vi "Update Preview Image.vi"(0 "Images (Dest)":T1, 2 "Buttons":T3, 3 "error in":errorcluster) -> (6 "Images (Out)":T1, 9 "error out":errorcluster)   [LabVIEW 2011]
uses:
  LCOS Images.ctl
  <vilib>/vision/Image Controls.llb/IMAQ Image.ctl
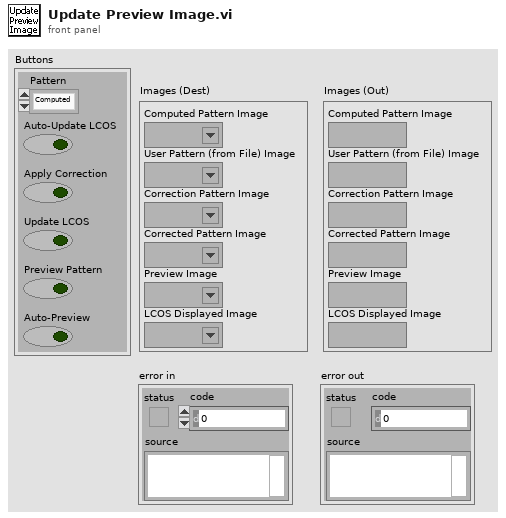
[diagram p1: front panel]
types:
  T1 = typedef "LCOS Images.ctl" = cluster{"Computed Pattern Image":T2, "User Pattern (from File) Image":T2, "Correction Pattern Image":T2, "Corrected Pattern Image":T2, "Preview Image":T2, "LCOS Displayed Image":T2}
  T2 = typedef "IMAQ Image.ctl" = refnum<image>
  T3 = cluster{"Pattern":enum16{"Computed", "From File", "Correction"}, "Auto-Update LCOS":bool, "Apply Correction":bool, "Update LCOS":bool, "Preview Pattern":bool, "Auto-Preview":bool}
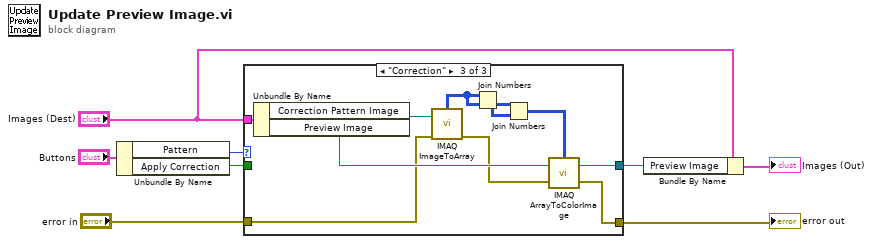
[diagram p0: block diagram]
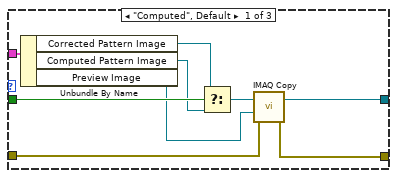
[diagram p2: hidden frame]
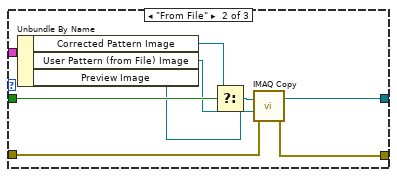
[diagram p3: hidden frame]
diagram:
  n1 = Unbundle By Name("Buttons") -> ("Pattern"=w7:enum16{"Computed", "From File", "Correction"}, "Apply Correction"=w6:bool)
  n2 = case shown="\"Correction\"" w7 {
    tunnel: w6 -> [w16 w25 _]
    tunnel: "Images (Dest)" -> [w17 w26 w36]
    tunnel: "error in" -> [w11 w20 w30]
    tunnel: [w10 w19 w27] -> w3
    tunnel: [w9 w18 w28] -> w1
    frame "Computed", Default {
      n3 = Unbundle By Name(w17) -> ("Corrected Pattern Image"=w15:T2, "Computed Pattern Image"=w14:T2, "Preview Image"=w12:T2)
      n4 = Select(t=w15, s=w16, f=w14) -> (s? t:f=w13:T2)
      n5 = call "IMAQ Copy"("error in (no error)"=w11, "Image Dst"=w12, "Image Src"=w13) -> ("error out"=w9:errorcluster, "Image Dst Out"=w10:T2)  [unwired: 3 in]
    }
    frame "From File" {
      n6 = Unbundle By Name(w26) -> ("Corrected Pattern Image"=w24:T2, "User Pattern (from File) Image"=w23:T2, "Preview Image"=w21:T2)
      n7 = Select(t=w24, s=w25, f=w23) -> (s? t:f=w22:T2)
      n8 = call "IMAQ Copy"("error in (no error)"=w20, "Image Dst"=w21, "Image Src"=w22) -> ("error out"=w18:errorcluster, "Image Dst Out"=w19:T2)  [unwired: 3 in]
    }
    frame "Correction" {
      n9 = Unbundle By Name(w36) -> ("Correction Pattern Image"=w35:T2, "Preview Image"=w31:T2)
      n10 = call "IMAQ ImageToArray"("error in (no error)"=w30, "Image"=w35) -> ("error out"=w29:errorcluster, "Image Pixels (U8)"=w34:u8[][])  [unwired: 2 in, 3 out]
      n11 = Join Numbers(hi=w34, lo=w34) -> ((hi.lo)=w33:u16[][])
      n12 = Join Numbers(hi=w34, lo=w33) -> ((hi.lo)=w32:u32[][])
      n13 = call "IMAQ ArrayToColorImage"("Image Pixels (U32)"=w32, "Image"=w31, "error in (no error)"=w29) -> ("Image Out"=w27:T2, "error out"=w28:errorcluster)  [unwired: 2 in]
    }
  }
  "error out" <- w1
  n14 = Bundle By Name(cluster="Images (Dest)", "Preview Image"=w3) -> (→"Images (Out)":T1)
